vi "Periodic Tasks.vi"(8 "error in":errorcluster) -> ()   [LabVIEW 2015]
doc: "This VI runs in parallel to other tasks. It can contain as many user-defined periodic loops as you need. These can carry out PID or other sorts of timed response."
uses:
  <vilib>/Analysis/baseanly.llb/Mean (DBL).vi
  Robot Global Data.vi
  <vilib>/Rock Robotics/Network Tables/NT Read Number.vi
  <vilib>/addons/control/pid/pid.llb/PID (DBL).vi
  <vilib>/Analysis/NI_AALBase.lvlib
  <vilib>/addons/control/pid/NI_PID_pid.lvlib
panel:
  out "8x filter":dbl(graph)
  in  "Arduino":u8
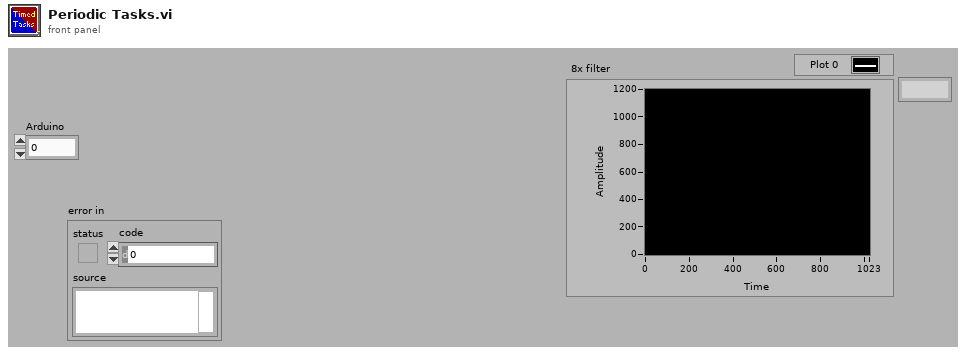
[diagram p1: front panel]
types:
  T1 = typedef "WPI_I2CDevRef.ctl" = cluster{"DevStatus":errorcluster, "Device Address":u8, "Handle":i32, "I2C Bus":T2}
  T2 = typedef "i2c_bus.ctl" = enum16{"I2C On-Board", "I2C MXP", "Invalid"}
  T3 = typedef "WPI_EncoderDevRef.ctl" = cluster{"DevStatus":errorcluster, "EncoderIndex":T4, "CounterIndex":T5, "DistancePerCount":dbl, "Decoding Type":T6}
  T4 = typedef "FPGA_EncoderIdx.ctl" = enum8{"Enc 0", "Enc 1", "Enc 2", "Enc 3", "Enc 4", "Enc 5", "Enc 6", "Enc 7", "Invalid"}
  T5 = typedef "FPGA_CounterCtrSystemIndex.ctl" = enum8{"Ctr 0", "Ctr 1", "Ctr 2", "Ctr 3", "Ctr 4", "Ctr 5", "Ctr 6", "Ctr 7", "Invalid"}
  T6 = typedef "WPI_EncoderType.ctl" = enum16{"1x", "2x", "4x"}
  T7 = cluster{"proportional gain (Kc)":dbl, "integral time (Ti, min)":dbl, "derivative time (Td, min)":dbl}
  T8 = typedef "WPI_MotorControlDeviceRef.ctl" = cluster{"DeviceStatus":errorcluster, "Type":T9, "PWM":cluster{"PWM Channel":T10, "DeadBand":T11}, "CAN":cluster{"Device Number":u8, "Control Mode":T12, "Semaphore":T13, "Max Vout":dbl, "TalonSRX Control Mode":T14}, "Invert":bool}
  T9 = typedef "WPI_MotorControlType.ctl" = enum16{"PWM", "CAN", "CANTalonSRX"}
  T10 = typedef "FPGA_DIOPWMChannel.ctl" = enum8{"PWM 0", "PWM 1", "PWM 2", "PWM 3", "PWM 4", "PWM 5", "PWM 6", "PWM 7", "PWM 8", "PWM 9", "PWM MXP 0", "PWM MXP 1", "PWM MXP 2", "PWM MXP 3", "PWM MXP 4", "PWM MXP 5", "PWM MXP 6", "PWM MXP 7", "PWM MXP 8", "PWM MXP 9", "Invalid"}
  T11 = typedef "WPI_PWMDeadband.ctl" = cluster{"Name":string, "maxPositivePwm":i32, "minPositivePwm":i32, "centerPwm":i32, "maxNegativePwm":i32, "minNegativePwm":i32, "angularRange":u16}
  T12 = typedef "WPI_CANJaguar_ControlMode.ctl" = enum8{"Percent VBus", "Current", "Speed", "Position", "Voltage"}
  T13 = typedef "Semaphore RefNum" = refnum<k1>
  T14 = typedef "WPI_CANTalonSRX_APIControlMode.ctl" = enum8{"Percent VBus", "Speed", "Position", "Slave", "Unchanged / Invalid", "Voltage Compensation", "Current", "Motion Profile"}
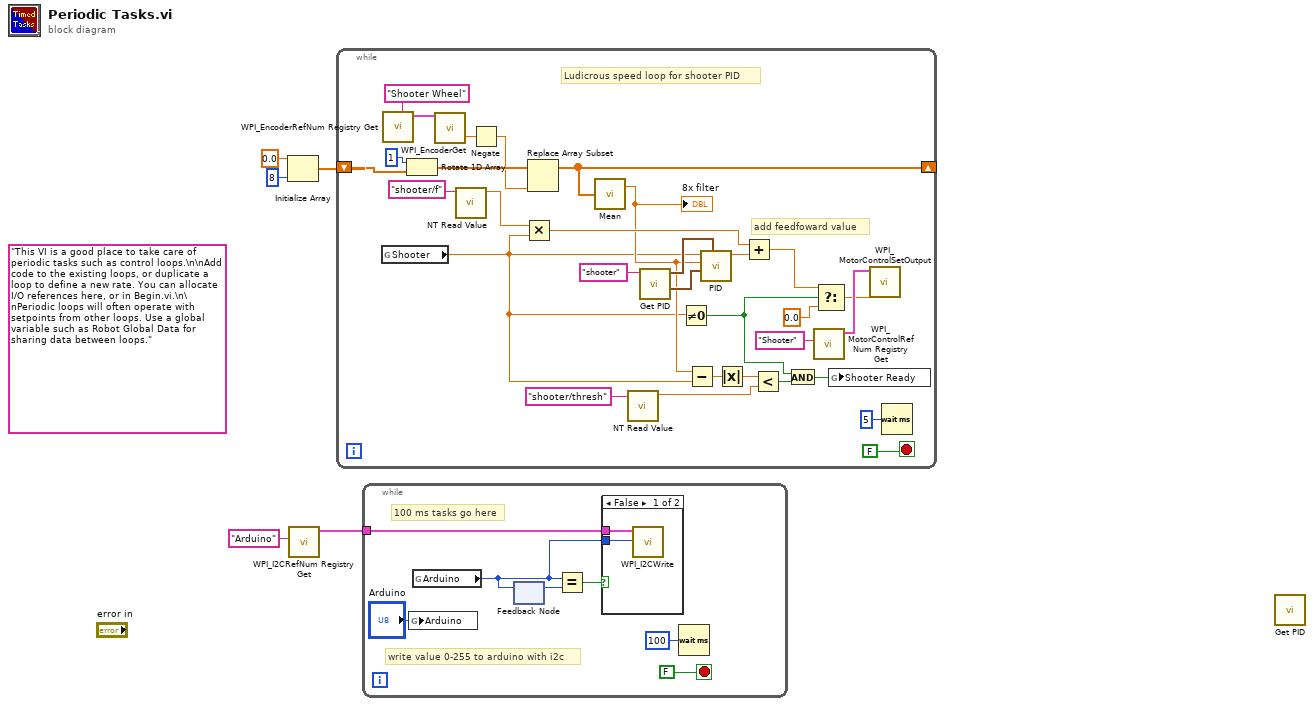
[diagram p0: block diagram]
diagram:
  (unwired) "This VI is a good place to take care of periodic tasks such as control loops.\n\nAdd code to the existing loops, or duplicate a loop to define a new rate. You can allocate I/O references here, or in Begin.vi.\n\nPeriodic loops will often operate with setpoints from other loops. Use a global variable such as Robot Global Data for sharing data between loops."
  n1 = Initialize Array(0.0 ("element"), 8 ("dimension size")) -> (w1:dbl[])
  n2 = call <vilib>:"WPI_I2CRefNum Registry Get.vi"("refnum name"="Arduino") -> ("I2CDevRef"=w5:T1)  [unwired: 9 in, 1 out]
  n3 = while {
    shift-right: [w27] -> _
    shift-left: w1 -> [w30]
    stop <- FALSE stop-if-true
    # "Ludicrous speed loop for shooter PID"
    # "add feedfoward value"
    n4 = global read "Robot Global Data.vi" "Shooter"() -> (w6:dbl)
    n5 = call <vilib>:"WPI_EncoderRefNum Registry Get.vi"("refnum name"="Shooter Wheel") -> ("EncoderDevRef"=w32:T3)  [unwired: 9 in, 1 out]
    n6 = Rotate 1D Array(1:w30, 2:1 ("n")) -> (0:w28:dbl[])
    n7 = call <vilib>:"WPI_EncoderGet.vi"("EncoderDevRef"=w32) -> ("Rate"=w25:dbl)  [unwired: 5 in, 5 out]
    n8 = call-poly <vilib>:"NT Read Value.vi"("Name"="shooter/f") -> ("Numeric"=w20:dbl)  [unwired: 9 in, 1 out]
    n9 = Negate(x=w25) -> (-x=w21:dbl)
    n10 = Multiply(x=w20, y=w6) -> (x*y=w19:dbl)
    n11 = Replace Array Subset(array=w28, new element=w21) -> (w27:dbl[])  [unwired: 1 in]
    n12 = call-poly <vilib>:"Mean.vi"("X"=w27) -> ("mean"=w14:dbl)  [unwired: 1 out]
    "8x filter" <- w14
    n13 = call-poly <vilib>:"NT Read Value.vi"("Name"="shooter/thresh") -> ("Numeric"=w10:dbl)  [unwired: 9 in, 1 out]
    n14 = call "Get PID.vi"("Subsystem"="shooter") -> ("PID Gains"=w22:T7, "output range"=w18:cluster{"output high":dbl, "output low":dbl})  [unwired: 8 in]
    n15 = Not Equal To 0?(x=w6) -> (x != 0?=w8:bool)
    n16 = Subtract(x=w14, y=w6) -> (x-y=w13:dbl)
    n17 = call-poly <vilib>:"PID.vi"("output range"=w18, "PID gains"=w22, "process variable"=w14, "setpoint"=w6) -> ("output"=w26:dbl)  [unwired: 6 in, 1 out]
    n18 = Absolute Value(x=w13) -> (abs(x)=w12:dbl)
    n19 = Add(x=w19, y=w26) -> (x+y=w17:dbl)
    n20 = Less?(x=w12, y=w10) -> (x < y?=w9:bool)
    n21 = And(x=w8, y=w9) -> (x .and. y?=w7:bool)
    n22 = call <vilib>:"WPI_MotorControlRefNum Registry Get.vi"("refnum name"="Shooter") -> ("MotorControlDevRef"=w33:T8)  [unwired: 9 in, 1 out]
    n23 = Select(t=w17, s=w8, f=0.0) -> (s? t:f=w16:dbl)
    n24 = global write "Robot Global Data.vi" "Shooter Ready"(w7) -> ()
    n25 = call <vilib>:"WPI_MotorControlSetOutput.vi"("Output"=w16, "MotorControlDevRef"=w33) -> ()  [unwired: 7 in, 3 out]
    n26 = Wait (ms)(milliseconds to wait=u32 5) -> ()  [unwired: 1 out]
  }
  n27 = while {
    tunnel: w5 -> [w40]
    stop <- FALSE stop-if-true
    # "write value 0-255 to arduino with i2c"
    # "100 ms tasks go here"
    n28 = global write "Robot Global Data.vi" "Arduino"("Arduino") -> ()
    n29 = global read "Robot Global Data.vi" "Arduino"() -> (w38:u8)
    n30 = feedback-in #1(w38) -> ()
    n31 = feedback #1() -> (w39:u8)  [unwired: 1 in]
    n32 = Equal?(x=w38, y=w39) -> (x = y?=w41:bool)
    n33 = case shown="False" w41 {
      tunnel: w40 -> [w45 _]
      tunnel: w38 -> [w44 _]
      frame False {
        n34 = call <vilib>:"WPI_I2CWrite.vi"("I2CRegister"=w44, "I2CDevRef"=w45) -> ()  [unwired: 8 in, 2 out]
      }
      frame True {
      }
    }
    n35 = Wait (ms)(milliseconds to wait=u32 100) -> ()  [unwired: 1 out]
  }
  n36 = call "Get PID.vi"() -> ()  [unwired: 9 in, 2 out]
